vi "CreateEventJSON.vi"(8 "error in (no error)":errorcluster, 10 "eventinfo":variant, 11 "type":string) -> (0 "error out":errorcluster, 3 "eventJSON":variant)   [LabVIEW 2018]
uses:
  <vilib>/LVH/i3 JSON/JSON Generation/Create Value Files/Create Value - Object.vi
  <vilib>/LVH/i3 JSON/JSON Generation/Add Object Parameter Files/Add Object Parameter - String.vi
  <vilib>/LVH/i3 JSON/JSON Generation/Add Object Parameter Files/Add Object Parameter - Object.vi
  <vilib>/LVH/i3 JSON/i3-json.lvlib
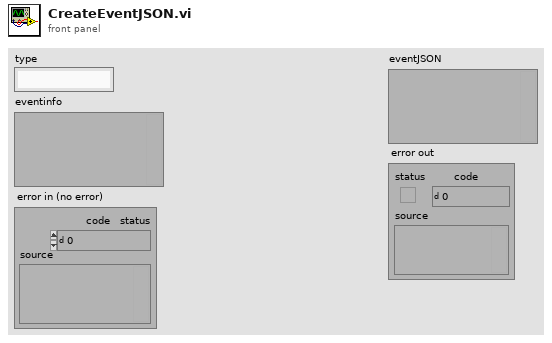
[diagram p1: front panel]
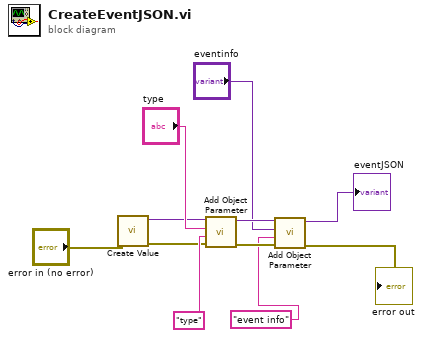
[diagram p0: block diagram]
diagram:
  n1 = call-poly <vilib>:"Create Value.vi"("error in (no error)"="error in (no error)") -> ("error out"=w9:errorcluster, "JSON Tree"=w8:variant)  [unwired: 9 in]
  n2 = call-poly <vilib>:"Add Object Parameter.vi"("error in (no error)"=w9, "Name"="type", "String"="type", "JSON Tree in (JSON Object)"=w8) -> ("error out"=w6:errorcluster, "JSON Tree out (JSON Object)"=w7:variant)  [unwired: 6 in]
  n3 = call-poly <vilib>:"Add Object Parameter.vi"("error in (no error)"=w6, "Name"="event info", "JSON Object"="eventinfo", "JSON Tree in (JSON Object)"=w7) -> ("error out"=→"error out":errorcluster, "JSON Tree out (JSON Object)"=→"eventJSON":variant)  [unwired: 6 in]
